vi "Toolkit Error Handling - VI Tree.vi"   [LabVIEW 2011]
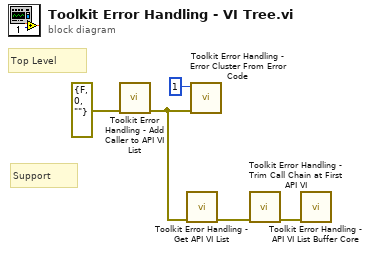
[diagram p0: block diagram]
diagram:
  # "Support"
  # "Top Level"
  n1 = call "Toolkit Error Handling - Add Caller to API VI List.vi"("error in"=errorcluster {"status"=FALSE, "code"=0, "source"=""}) -> ("error out"=w3:errorcluster)  [unwired: 10 in]
  n2 = call "Toolkit Error Handling - Get API VI List.vi"("error in (no error)"=w3) -> ("error out"=w5:errorcluster)  [unwired: 9 in, 1 out]
  n3 = call "Toolkit Error Handling - Error Cluster From Error Code.vi"("error in"=w3, "error code (0)"=1) -> ()  [unwired: 7 in, 1 out]
  n4 = call "Toolkit Error Handling - Trim Call Chain at First API VI.vi"("error in (no error)"=w5) -> ("error out"=w2:errorcluster)  [unwired: 9 in, 1 out]
  n5 = call "Toolkit Error Handling - API VI List Buffer Core.vi"("error in (no error)"=w2) -> ()  [unwired: 9 in, 2 out]
